vi "Initialize Setting.vi"(7 "Depth":T1 items=["WRITE AREA", "RUNNING AREA", "SAVE AREA"], 8 "error in (no error)":errorcluster {"code" format="%.0x"}, 10 "Target":T2 items=["PROGRAM 0", "PROGRAM 1", "PROGRAM 2", "PROGRAM 3", "PROGRAM 4", "PROGRAM 5", "PROGRAM 6", "PROGRAM 7", "PROGRAM 8", "PROGRAM 9", "PROGRAM 10", "PROGRAM 11", "PROGRAM 12", "PROGRAM 13", "PROGRAM 14", "PROGRAM 15"], 11 "Device ID (0)":i32) -> (0 "error out":errorcluster {"code" format="%.0x"}, 3 "Device ID out":i32)   [LabVIEW 2020, in "KEYENCE LJ-X8000A.lvlib"]
doc: "This function initializes the setting of the area specified as the initialization target."
uses:
  KEYENCE LJ-X8000A.lvlib
  Constants/Init Setting Target.ctl
  Constants/Setting Depth.ctl
panel:
  # "(c) 2019 KEYENCE CORPORATION.  ALL RIGHTS RESERVED."
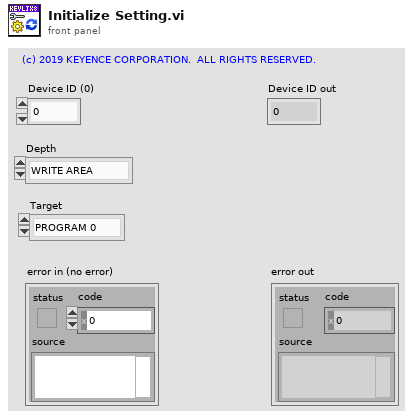
[diagram p1: front panel]
types:
  T1 = typedef "KEYENCE LJ-X8000A.lvlib/Setting Depth.ctl" = u8
  T2 = typedef "KEYENCE LJ-X8000A.lvlib/Init Setting Target.ctl" = u8
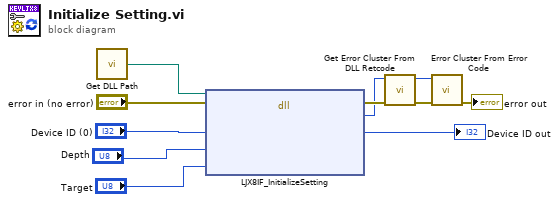
[diagram p0: block diagram]
diagram:
  n1 = call "Get DLL Path.vi"() -> ("DLL Path"=w6:path)  [unwired: 3 in]
  n2 = dll-call lib="C:/Program Files (x86)/National Instruments/LabVIEW 2018/instr.lib/KEYENCE LJ-X8000/LJX8_IF.*" fn="LJX8IF_InitializeSetting"(path in=w6, error in="error in (no error)", "lDeviceId"="Device ID (0)", "byDepth"="Depth", "byTarget"="Target") -> (error out=w4:errorcluster, "lRetCode"=w3:i32, "lDeviceId"=→"Device ID out":i32)  [unwired: 3 in, 1 out]
  n3 = call "Get Error Cluster From DLL Retcode.vi"("error in (no error)"=w4, "DLL Return Code"=w3) -> ("error out"=w5:errorcluster, "VI Error Code"=w1:i32)  [unwired: 8 in]
  n4 = call <vilib>:"Error Cluster From Error Code.vi"("error in (no error)"=w5, "error code (0)"=w1) -> ("error out"=→"error out":errorcluster)  [unwired: 7 in]
